vi "SubVI_SVM_test_Craik.vi"(4 "Alpha (idx)":dbl[][](array[numeric]), 5 "Testing Data":dbl[][](array[numeric]), 6 "Label (idx)":dbl[][](array[numeric]), 7 "training (idx)":dbl[][](array[numeric]), 9 "Linear or Gaussian":string, 10 "b":dbl, 11 "w":dbl[][](array[numeric])) -> (3 "Prediction":dbl[][](array[numeric]))   [LabVIEW 2020]
uses:
  <vilib>/Analysis/baseanly.llb/Real A x B.vi
  <vilib>/Analysis/Matrix/Numeric/Multiply/Multiply - RM,R.vi
  <vilib>/Analysis/Matrix/Numeric/Subtract/Subtract - RM,RM.vi
  <vilib>/Analysis/Matrix/Numeric/Add/Add - RM,RM.vi
  <vilib>/Analysis/Matrix/Numeric/Conversions/Matrix To Array - RM.vi
  <vilib>/Analysis/Matrix/Numeric/Add/Add (Elementwise) - RM,R.vi
  <vilib>/Analysis/NI_AALBase.lvlib
  <vilib>/Analysis/Matrix/NI_Matrix.lvlib
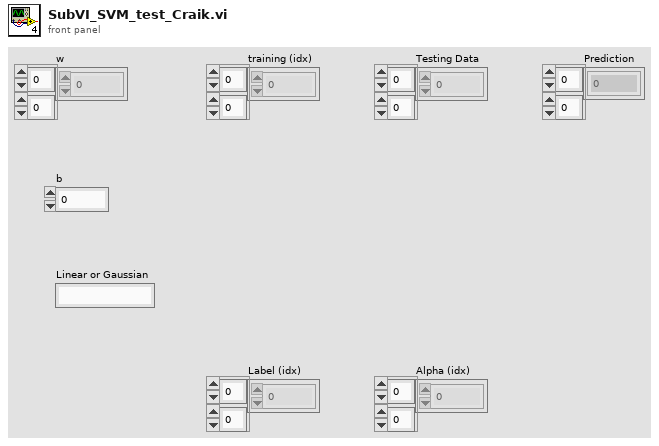
[diagram p1: front panel]
types:
  T1 = typedef "NI_Matrix.lvlib/RealMatrix.ctl" = dbl[][]
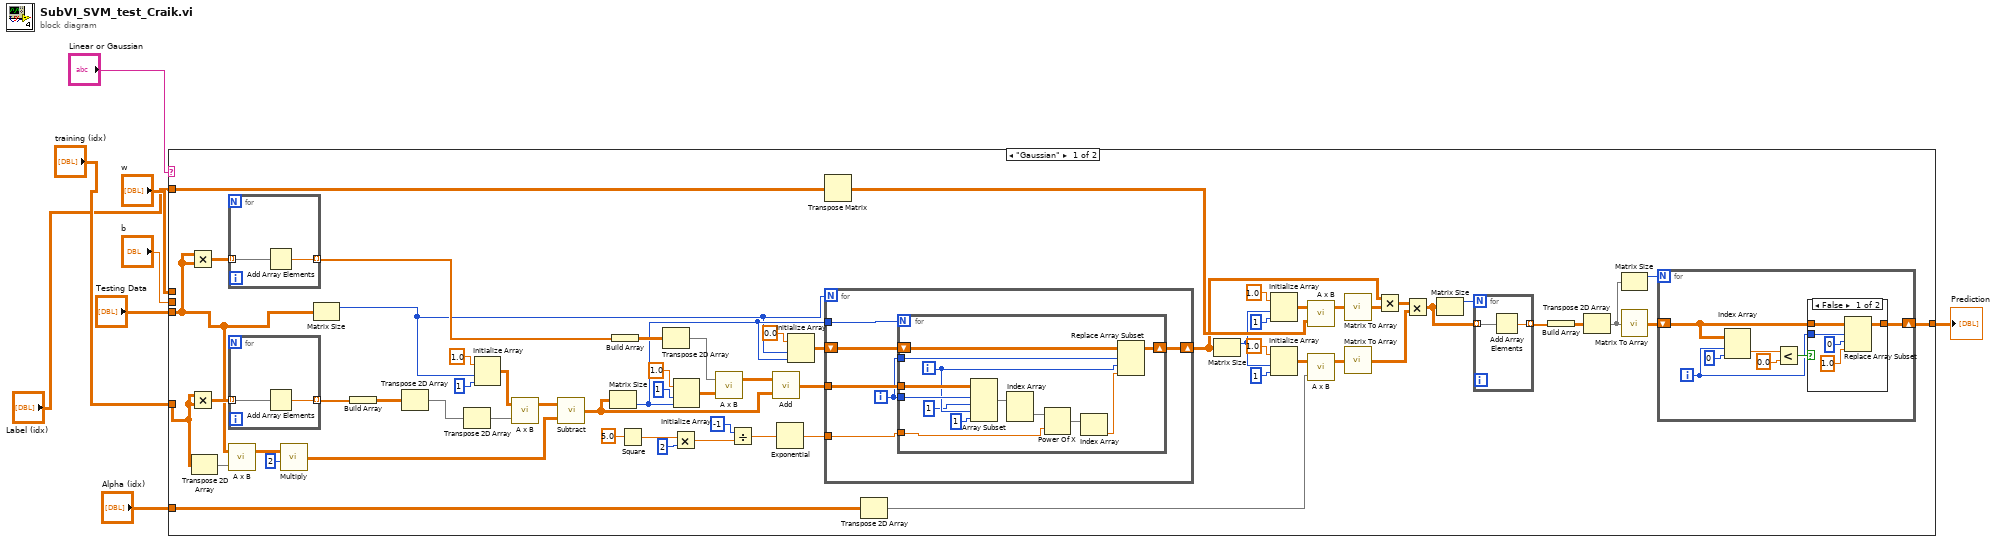
[diagram p0: block diagram]
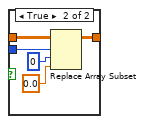
[diagram p2: hidden frame]
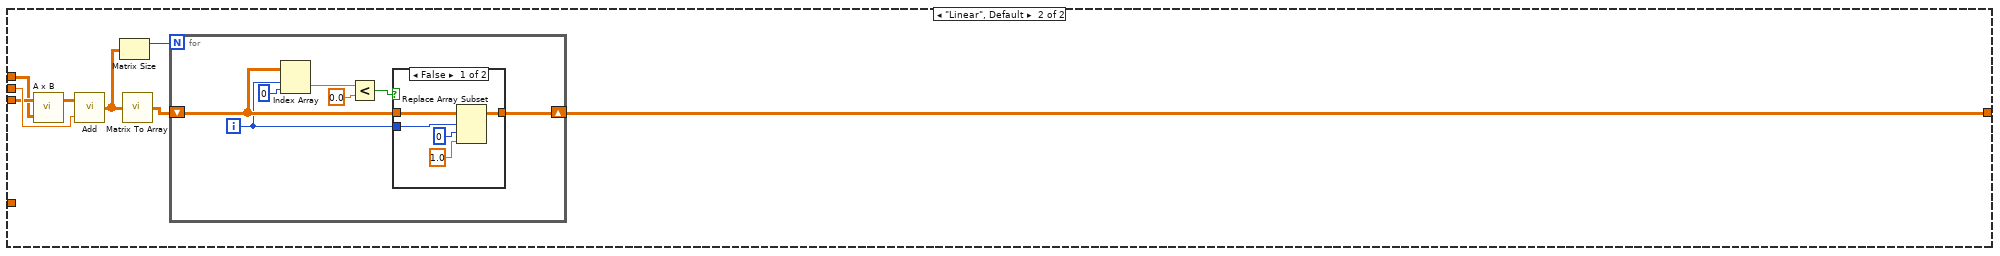
[diagram p3: hidden frame]
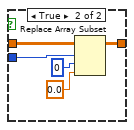
[diagram p4: hidden frame]
diagram:
  n1 = case shown="\"Gaussian\"" "Linear or Gaussian" {
    tunnel: "Testing Data" -> [w9 w113]
    tunnel: "b" -> [_ w118]
    tunnel: [w12 w114] -> w5
    tunnel: "Label (idx)" -> [w37 _]
    tunnel: "training (idx)" -> [w33 _]
    tunnel: "Alpha (idx)" -> [w28 _]
    tunnel: "w" -> [_ w112]
    frame "Gaussian" {
      n2 = Multiply(x=w9, y=w9) -> (x*y=w46:dbl[][])
      n3 = Multiply(x=w33, y=w33) -> (x*y=w11:dbl[][])
      n4 = Transpose 2D Array(2D array=w33) -> (transposed array=w51:dbl[][])
      n5 = for {
        tunnel: w46 -> [w90] mode=indexing
        tunnel: [w89] -> w47 mode=indexing
        n6 = Add Array Elements(numeric array=w90) -> (sum=w89:dbl)
      }
      n7 = for {
        tunnel: w11 -> [w110] mode=indexing
        tunnel: [w111] -> w49 mode=indexing
        n8 = Add Array Elements(numeric array=w110) -> (sum=w111:dbl)
      }
      n9 = call-poly <vilib>:"A x B.vi"("B"=w51, "A"=w9) -> ("A x B"=w52:T1)  [unwired: 1 out]
      n10 = call-poly <vilib>:"Multiply.vi"("Real Scalar c"=2, "Real Matrix A"=w52) -> ("A * c"=w57:T1)
      n11 = Matrix Size(0:w9) -> (1:w10:i32)  [unwired: 1 out]
      n12 = Build Array(w49) -> (w50:dbl[][])
      n13 = Transpose 2D Array(2D array=w50) -> (transposed array=w59:dbl[][])
      n14 = Transpose 2D Array(2D array=w59) -> (transposed array=w56:dbl[][])
      n15 = Initialize Array(1.0 ("element"), w10, 1 ("dimension size")) -> (w60:dbl[][])
      n16 = call-poly <vilib>:"A x B.vi"("B"=w56, "A"=w60) -> ("A x B"=w58:T1)  [unwired: 1 out]
      n17 = call-poly <vilib>:"Subtract.vi"("Real Matrix B"=w57, "Real Matrix A"=w58) -> ("A - B"=w40:T1)
      n18 = Matrix Size(0:w40) -> (2:w38:i32)  [unwired: 1 out]
      n19 = Build Array(w47) -> (w48:dbl[][])
      n20 = Square(x=5.0) -> (x^2=w61:dbl)
      n21 = Transpose 2D Array(2D array=w48) -> (transposed array=w43:dbl[][])
      n22 = Multiply(x=w61, y=2) -> (x*y=w64:dbl)
      n23 = Initialize Array(1.0 ("element"), 1 ("dimension size"), w38) -> (w41:dbl[][])
      n24 = call-poly <vilib>:"A x B.vi"("B"=w41, "A"=w43) -> ("A x B"=w44:T1)  [unwired: 1 out]
      n25 = Divide(x=-1, y=w64) -> (x/y=w65:dbl)
      n26 = call-poly <vilib>:"Add.vi"("Real Matrix B"=w40, "Real Matrix A"=w44) -> ("A + B"=w67:T1)
      n27 = Exponential(1:w65) -> (0:w66:dbl)
      n28 = Initialize Array(0.0 ("element"), w10, w38) -> (w69:dbl[][])
      n29 = Transpose Matrix(1:w37) -> (0:w32:dbl[][])
      n30 = for {
        N: w10 -> [_]
        tunnel: w66 -> [w93]
        tunnel: w67 -> [w95]
        shift-right: [w92] -> w19
        shift-left: w69 -> [w96]
        tunnel: w38 -> [w91]
        i -> [w94]
        n31 = for {
          N: w91 -> [_]
          tunnel: w94 -> [w108]
          tunnel: w95 -> [w107]
          tunnel: w94 -> [w106]
          tunnel: w93 -> [w102]
          shift-right: [w103] -> w92
          shift-left: w96 -> [w109]
          i -> [w101]
          n32 = Array Subset(array=w107, index (row)=w106, length (row)=1 ("length"), index (col)=w101, length (col)=1 ("length")) -> (w98:T1)
          n33 = Index Array(array=w98) -> (element=w97:dbl[])  [unwired: 2 in]
          n34 = Power Of X(1:w102, 2:w97) -> (0:w105:dbl[])
          n35 = Index Array(array=w105) -> (element=w104:dbl)  [unwired: 1 in]
          n36 = Replace Array Subset(array=w109, new element=w104, index (row)=w108, index (col)=w101) -> (w103:dbl[][])
        }
      }
      n37 = Transpose 2D Array(2D array=w28) -> (transposed array=w16:dbl[][])
      n38 = Matrix Size(0:w19) -> (1:w18:i32)  [unwired: 1 out]
      n39 = Initialize Array(1.0 ("element"), w18, 1 ("dimension size")) -> (w35:dbl[][])
      n40 = Initialize Array(1.0 ("element"), w18, 1 ("dimension size")) -> (w17:dbl[][])
      n41 = call-poly <vilib>:"A x B.vi"("B"=w32, "A"=w35) -> ("A x B"=w27:T1)  [unwired: 1 out]
      n42 = call-poly <vilib>:"A x B.vi"("B"=w16, "A"=w17) -> ("A x B"=w29:T1)  [unwired: 1 out]
      n43 = call-poly <vilib>:"Matrix To Array.vi"("Real Matrix"=w27) -> ("Real 2D Array"=w20:dbl[][])
      n44 = call-poly <vilib>:"Matrix To Array.vi"("Real Matrix"=w29) -> ("Real 2D Array"=w25:dbl[][])
      n45 = Multiply ("Multiply.vi")(x=w19, y=w20) -> (x*y=w26:dbl[][])
      n46 = Multiply ("Multiply.vi")(x=w26, y=w25) -> (x*y=w23:dbl[][])
      n47 = Matrix Size(0:w23) -> (1:w22:i32)  [unwired: 1 out]
      n48 = for {
        N: w22 -> [_]
        tunnel: w23 -> [w88] mode=indexing
        tunnel: [w87] -> w24 mode=indexing
        n49 = Add Array Elements(numeric array=w88) -> (sum=w87:dbl)
      }
      n50 = Build Array(w24) -> (w21:dbl[][])
      n51 = Transpose 2D Array(2D array=w21) -> (transposed array=w13:dbl[][])
      n52 = Matrix Size(0:w13) -> (1:w14:i32)  [unwired: 1 out]
      n53 = call-poly <vilib>:"Matrix To Array.vi"("Real Matrix"=w13) -> ("Real 2D Array"=w15:dbl[][])
      n54 = for {
        N: w14 -> [_]
        shift-right: [w70] -> w12
        shift-left: w15 -> [w72]
        i -> [w71]
        n55 = Index Array(array=w72, index (row)=w71, index (col)=0 ("disabled index (col)")) -> (element=w75:dbl)
        n56 = Less?(x=w75, y=0.0) -> (x < y?=w73:bool)
        n57 = case shown="False" w73 {
          tunnel: w72 -> [w78 w86]
          tunnel: w71 -> [w79 w85]
          tunnel: [w77 w82] -> w70
          frame False {
            n58 = Replace Array Subset(array=w78, new element=1.0 ("new element/subarray"), index (row)=w79, index (col)=0 ("disabled index (col)")) -> (w77:dbl[][])
          }
          frame True {
            n59 = Replace Array Subset(array=w86, new element=0.0 ("new element/subarray"), index (row)=w85, index (col)=0 ("disabled index (col)")) -> (w82:dbl[][])
          }
        }
      }
    }
    frame "Linear", Default {
      n60 = call-poly <vilib>:"A x B.vi"("B"=w112, "A"=w113) -> ("A x B"=w119:T1)  [unwired: 1 out]
      n61 = call-poly <vilib>:"Add.vi"("Real Scalar c"=w118, "Real Matrix A"=w119) -> ("A + c"=w116:T1)
      n62 = Matrix Size(0:w116) -> (1:w115:i32)  [unwired: 1 out]
      n63 = call-poly <vilib>:"Matrix To Array.vi"("Real Matrix"=w116) -> ("Real 2D Array"=w117:dbl[][])
      n64 = for {
        N: w115 -> [_]
        shift-right: [w120] -> w114
        shift-left: w117 -> [w122]
        i -> [w121]
        n65 = Index Array(array=w122, index (row)=w121, index (col)=0 ("disabled index (col)")) -> (element=w125:dbl)
        n66 = Less?(x=w125, y=0.0) -> (x < y?=w123:bool)
        n67 = case shown="False" w123 {
          tunnel: w122 -> [w128 w136]
          tunnel: w121 -> [w129 w135]
          tunnel: [w127 w132] -> w120
          frame False {
            n68 = Replace Array Subset(array=w128, new element=1.0 ("new element/subarray"), index (row)=w129, index (col)=0 ("disabled index (col)")) -> (w127:dbl[][])
          }
          frame True {
            n69 = Replace Array Subset(array=w136, new element=0.0 ("new element/subarray"), index (row)=w135, index (col)=0 ("disabled index (col)")) -> (w132:dbl[][])
          }
        }
      }
    }
  }
  "Prediction" <- w5
